vi "Pos_Calculate Random Location.vi"(8 "Error":errorcluster, 9 "Window Size":i16, 10 "Border":i16, 11 "Max Size":i16) -> (0 "Error Out":errorcluster, 2 "Bottom Right Out":i16, 3 "Top Left Out":i16)   [LabVIEW 2024]
uses:
  <vilib>/numeric/Random Number (Range) I64.vi
  <vilib>/numeric/sub_Random U32.vi
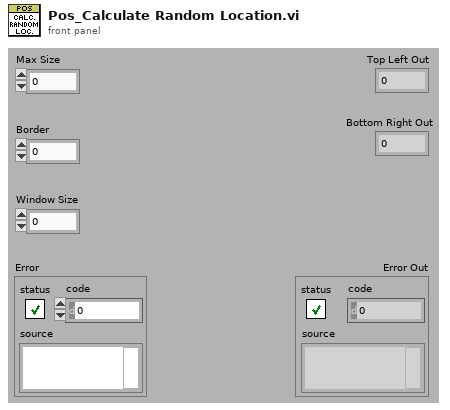
[diagram p1: front panel]
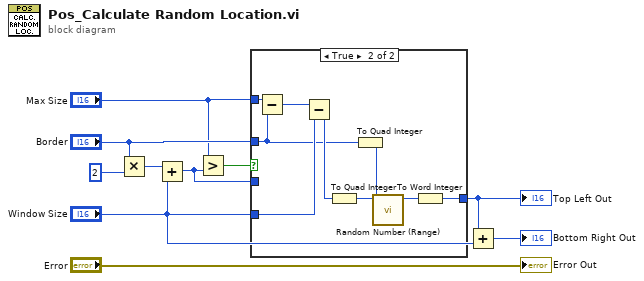
[diagram p0: block diagram]
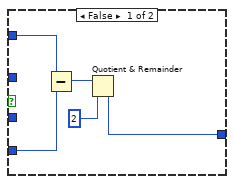
[diagram p2: hidden frame]
diagram:
  n1 = Multiply(x="Border", y=i16 2) -> (x*y=w8:i16)
  n2 = Add(x=w8, y="Window Size") -> (x+y=w4:i16)
  n3 = Greater?(x="Max Size", y=w4) -> (0:w7:bool)
  n4 = case shown="True" w7 {
    tunnel: "Border" -> [_ w19]
    tunnel: "Max Size" -> [w15 w24]
    tunnel: "Window Size" -> [w14 w22]
    tunnel: [w11 w21] -> w2
    tunnel: w4 -> [_ _]
    frame False {
      n5 = Subtract(x=w15, y=w14) -> (x-y=w13:i16)
      n6 = Quotient & Remainder(x=w13, y=i16 2) -> (floor(x/y)=w11:i16)  [unwired: 1 out]
    }
    frame True {
      n7 = Subtract(x=w24, y=w19) -> (x-y=w23:i16)
      n8 = Subtract(x=w23, y=w22) -> (x-y=w20:i16)
      n9 = To Quad Integer(1:w20) -> (0:w17:i64)
      n10 = To Quad Integer(1:w19) -> (0:w18:i64)
      n11 = call-poly <vilib>:"Random Number (Range).vi"("lower bound (-100)"=w18, "upper bound (100)"=w17) -> ("number"=w16:i64)  [unwired: 9 in]
      n12 = To Word Integer(number=w16) -> (16bit integer=w21:i16)
    }
  }
  "Top Left Out" <- w2
  n13 = Add(x=w2, y="Window Size") -> (x+y=→"Bottom Right Out":i16)
  "Error Out" <- "Error"
